vi "Teleop.vi"(10 "Match Info":T1={"Autonomous Elapsed Seconds"=0.0, "TeleOp Elapsed Seconds"=0.0, "Disabled Elapsed Seconds"=0.0, "Visited Autonomous"=FALSE, "Visited TeleOp"=FALSE, "Visited Disabled"=FALSE, "Autonomous Settings"={"Autonomous Style"=enum."Independent", "VI Refnum"=refnum}}, 11 "Call Context":T2) -> ()   [LabVIEW 2017]
doc: "This VI is called for each enabled TeleOp packet received from the DS. It is typically used to read from joysticks and other inputs and update I/O or setpoints for timed control loops. It should complete and return within 20 milliseconds or risk missing DS packets."
uses:
  <vilib>/Rock Robotics/WPI/DriverStation/WPI_DriverStationDerivedRobotMode.ctl
  <vilib>/Rock Robotics/WPI/DriverStation/WPI_DriverStationMatch Info.ctl
  <vilib>/Rock Robotics/WPI/Utilities/WPI_GetSetVariantRefNum.vi
  <vilib>/Rock Robotics/Network Tables/NT Write Boolean Array.vi
  <vilib>/Rock Robotics/Network Tables/NT Write Numeric Array.vi
panel:
  out "LeftJoystick":cluster{"X":dbl, "Y":dbl}[](graph)
  out "RightJoystick":cluster{"X":dbl, "Y":dbl}[](graph)
  out "Waveform Chart":cluster{i16, i16, i16, i16, i16}(graph)
  in  "toFreestyle":bool
  in  "toDriveDistance":bool
  in  "toTurnAngle":bool
  in  "toDoNothing":bool
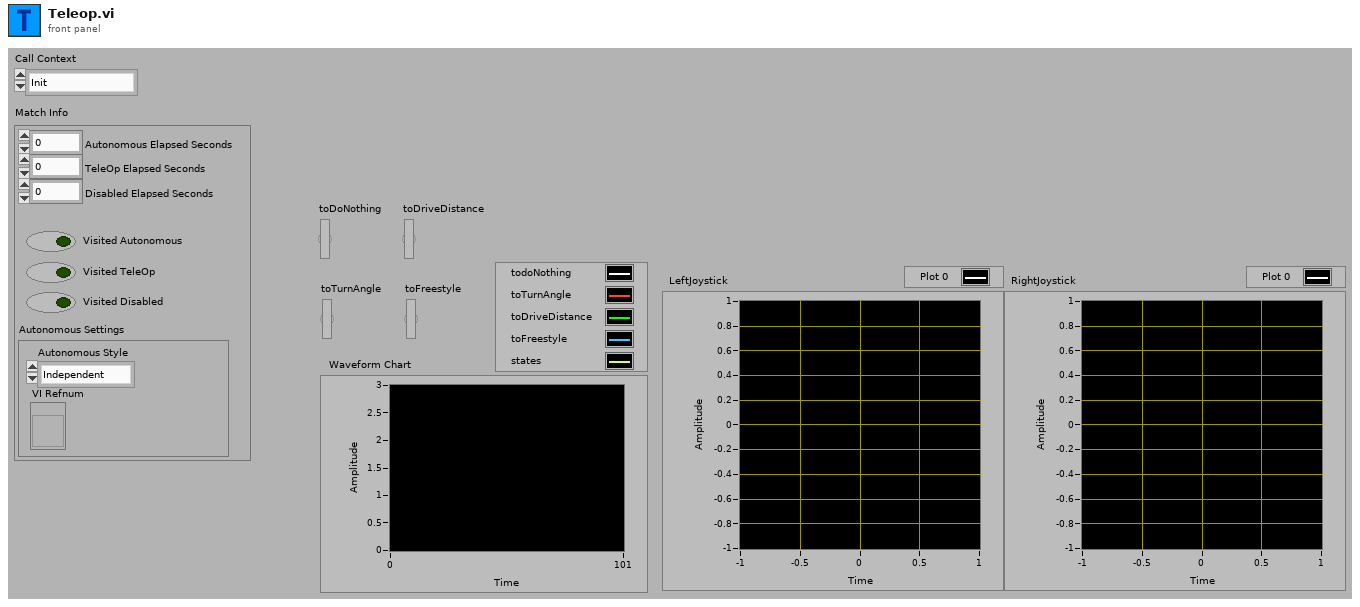
[diagram p1: front panel]
types:
  T1 = typedef "WPI_DriverStationMatch Info.ctl" = cluster{"Autonomous Elapsed Seconds":dbl, "TeleOp Elapsed Seconds":dbl, "Disabled Elapsed Seconds":dbl, "Visited Autonomous":bool, "Visited TeleOp":bool, "Visited Disabled":bool, "Autonomous Settings":cluster{"Autonomous Style":enum16{"Iterative", "Independent"}, "VI Refnum":refnum<vi>}}
  T2 = typedef "WPI_DriverStationDerivedRobotMode.ctl" = enum16{"Init", "Execute", "Stop"}
  T3 = typedef "WPI_JoystickDevRef.ctl" = cluster{"Device":T4}
  T4 = typedef "WPI_JoystickDeviceEnum.ctl" = enum16{"USB 0", "USB 1", "USB 2", "USB 3", "USB 4", "USB 5"}
  T5 = typedef "Command Status Info.ctl" = cluster{"Name":string, "Status":T6, "notifier out":T7}
  T6 = typedef "Completion Status.ctl" = enum16{"Successful", "Aborted", "Incomplete"}
  T7 = typedef "Completion Notifier.ctl" = refnum<notifier>
  T8 = typedef "driveLogicStates.ctl" = enum16{"doNothing", "driveDistance", "turnAngle", "freestyle", "guidedDrive", "approachingElement"}
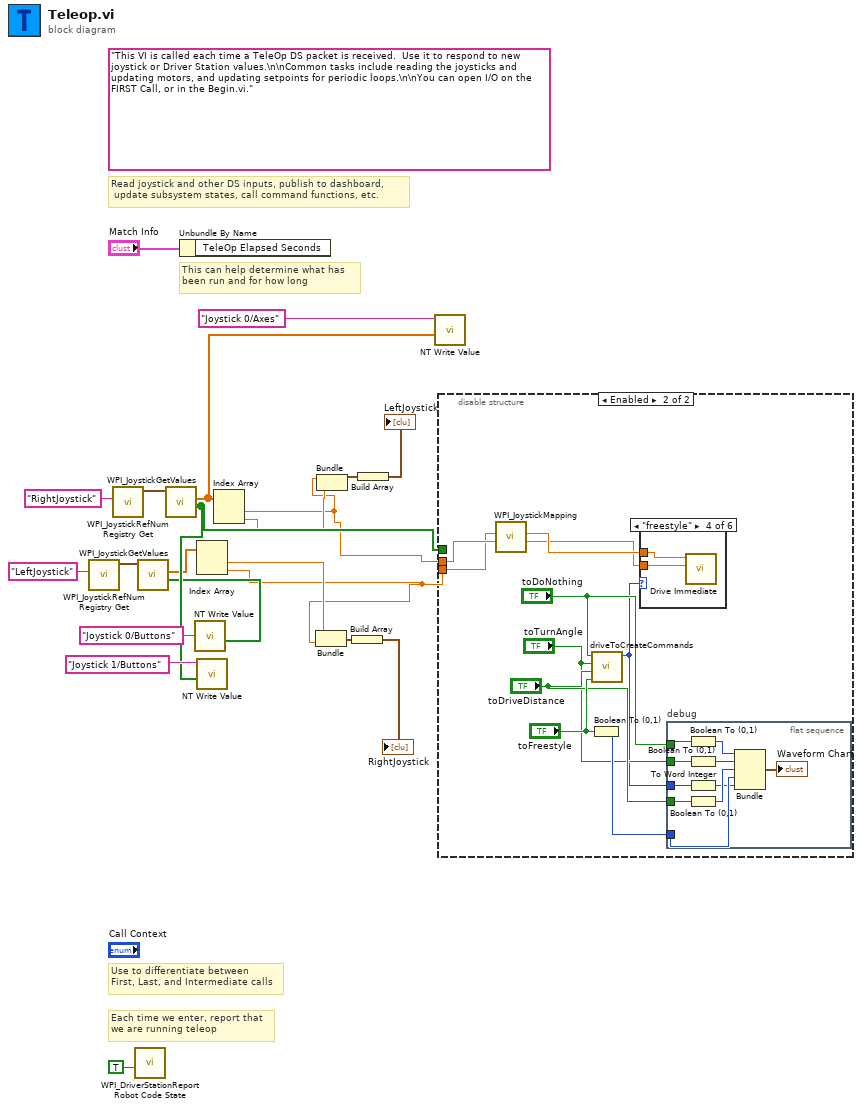
[diagram p0: block diagram]
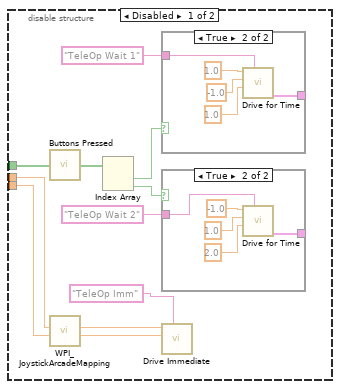
[diagram p2: hidden frame]
diagram:
  (unwired) "This VI is called each time a TeleOp DS packet is received.  Use it to respond to new joystick or Driver Station values.\n\nCommon tasks include reading the joysticks and updating motors, and updating setpoints for periodic loops.\n\nYou can open I/O on the FIRST Call, or in the Begin.vi."
  # "Read joystick and other DS inputs, publish to dashboard,\n update subsystem states, call command functions, etc."
  # "Each time we enter, report that\nwe are running teleop"
  # "Use to differentiate between\nFirst, Last, and Intermediate calls"
  # "This can help determine what has\nbeen run and for how long"
  n1 = call <vilib>:"WPI_JoystickRefNum Registry Get.vi"("refnum name"="LeftJoystick") -> ("JoystickDevRef"=w12:T3)  [unwired: 1 in, 9 out]
  n2 = call <vilib>:"WPI_JoystickRefNum Registry Get.vi"("refnum name"="RightJoystick") -> ("JoystickDevRef"=w18:T3)  [unwired: 1 in, 9 out]
  n3 = call <vilib>:"WPI_DriverStationReport Robot Code State.vi"("TeleOp"=TRUE ("Autonomous")) -> ()  [unwired: 10 in, 1 out]
  n4 = call <vilib>:"WPI_JoystickGetValues.vi"("JoystickDevRef"=w12) -> ("Buttons"=w10:bool[], "Axes"=w11:dbl[])  [unwired: 6 in, 3 out]
  n5 = call <vilib>:"WPI_JoystickGetValues.vi"("JoystickDevRef"=w18) -> ("Buttons"=w16:bool[], "Axes"=w15:dbl[])  [unwired: 6 in, 3 out]
  n6 = Unbundle By Name("Match Info") -> ()  [unwired: 1 out]
  n7 = call-poly <vilib>:"NT Write Value.vi"("Boolean Array"=w10, "Name"="Joystick 0/Buttons") -> ()  [unwired: 9 in, 1 out]
  n8 = Index Array(array=w11) -> (element #1=w3:dbl, element #2=w2:dbl)  [unwired: 2 in]
  n9 = call-poly <vilib>:"NT Write Value.vi"("Boolean Array"=w16, "Name"="Joystick 1/Buttons") -> ()  [unwired: 9 in, 1 out]
  n10 = Index Array(array=w15) -> (element #1=w1:dbl, element #2=w4:dbl)  [unwired: 2 in]
  n11 = Bundle("upper limit"=w3, "upper limit"=w2) -> (w8:cluster{"upper limit":dbl, "upper limit":dbl})  [unwired: 1 in]
  n12 = Bundle("upper limit"=w1, "upper limit"=w4) -> (w6:cluster{"upper limit":dbl, "upper limit":dbl})  [unwired: 1 in]
  n13 = Build Array(w8) -> (→"RightJoystick":cluster{"upper limit":dbl, "upper limit":dbl}[])
  n14 = Build Array(w6) -> (→"LeftJoystick":cluster{"upper limit":dbl, "upper limit":dbl}[])
  n15 = call-poly <vilib>:"NT Write Value.vi"("Numeric Array"=w15, "Name"="Joystick 0/Axes") -> ()  [unwired: 9 in, 1 out]
  n16 = disable-structure shown="Enabled" {
    disable-tunnel: w1 -> [w24 w44]
    disable-tunnel: w2 -> [w23 w43]
    disable-tunnel: w16 -> [w22 _]
    frame Disabled {
      n17 = call "Buttons Pressed.vi"("Button Values"=w22) -> ("Button Presses"=w29:bool[])
      n18 = call <vilib>:"WPI_JoystickArcadeMapping.vi"("Y axis value"=w23, "X axis value"=w24) -> ("Right Motor Value"=w25:dbl, "Left Motor Value"=w26:dbl)  [unwired: 8 in]
      n19 = Index Array(array=w29) -> (element #1=w28:bool, element #2=w27:bool)  [unwired: 2 in]
      n20 = case shown="True" w28 {
        tunnel: [_ w41] -> _
        tunnel: "TeleOp Wait 1" ("Description") -> [_ w40]
        frame False {
        }
        frame True {
          n21 = call "Drive for Time.vi"("Description"=w40, "Seconds"=1.0, "Right Speed"=-1.0, "Left Speed"=1.0) -> ("Command Info Out"=w41:T5)  [unwired: 6 in, 1 out]
        }
      }
      n22 = case shown="True" w27 {
        tunnel: [_ w35] -> _
        tunnel: "TeleOp Wait 2" ("Description") -> [_ w34]
        frame False {
        }
        frame True {
          n23 = call "Drive for Time.vi"("Description"=w34, "Seconds"=2.0, "Right Speed"=1.0, "Left Speed"=-1.0) -> ("Command Info Out"=w35:T5)  [unwired: 6 in, 1 out]
        }
      }
      n24 = call "Drive Immediate.vi"("Description"="TeleOp Imm", "Right Setpoint"=w25, "Left Setpoint"=w26) -> ()  [unwired: 8 in, 1 out]
    }
    frame Enabled {
      n25 = call-poly <vilib>:"WPI_JoystickMapping.vi"("Y axis value"=w44, "X axis value"=w43) -> ("Right Motor Value"=w45:dbl, "Left Motor Value"=w46:dbl)  [unwired: 8 in]
      n26 = Boolean To (0,1)(Boolean="toFreestyle") -> (0, 1=w51:i16)
      n27 = call "driveToCreateCommands.vi"("toFreestyle"="toFreestyle", "toDriveDistance"="toDriveDistance", "toTurnAngle"="toTurnAngle", "toDoNothing"="toDoNothing") -> ("Current state"=w47:T8)  [unwired: 7 in]
      n28 = case shown="\"freestyle\"" w47 {
        tunnel: w46 -> [_ _ _ w63 _ _]
        tunnel: w45 -> [_ _ _ w64 _ _]
        frame "doNothing", Default {
        }
        frame "driveDistance" {
        }
        frame "turnAngle" {
        }
        frame "freestyle" {
          n29 = call "Drive Immediate.vi"("Right Setpoint"=w64, "Left Setpoint"=w63) -> ()  [unwired: 9 in, 1 out]
        }
        frame "guidedDrive" {
        }
        frame "approachingElement" {
        }
      }
      n30 = flat-sequence "debug" {
        tunnel: w51 -> [w62]
        tunnel: "toDriveDistance" -> [w61]
        tunnel: "toTurnAngle" -> [w60]
        tunnel: "toDoNothing" -> [w59]
        tunnel: w47 -> [w53]
        frame #0 {
          n31 = Boolean To (0,1)(Boolean=w59) -> (0, 1=w56:i16)
          n32 = Boolean To (0,1)(Boolean=w60) -> (0, 1=w57:i16)
          n33 = To Word Integer(number=w53) -> (16bit integer=w54:i16)
          n34 = Boolean To (0,1)(Boolean=w61) -> (0, 1=w58:i16)
          n35 = Bundle(w56, w57, w58, w62, w54) -> (→"Waveform Chart":cluster{i16, i16, i16, i16, i16})  [unwired: 1 in]
        }
      }
    }
  }
